vi "Extract Files HTML from SubFolder (Row).vi"(8 "error in (no error)":errorcluster, 10 "SearchFolder":string, 11 "Folder_Mgmt in":refnum<class "Folder_Mgmt.lvclass">) -> (0 "error out":errorcluster, 2 "FolderFiles (Row)":string[](array[string]), 3 "Folder_Mgmt out":refnum<class "Folder_Mgmt.lvclass">)   [LabVIEW 2016, in "Folder_Mgmt.lvclass"]
uses:
  Folder_Mgmt.lvclass
  Folder_Mgmt.lvclass/Folder_Mgmt.ctl
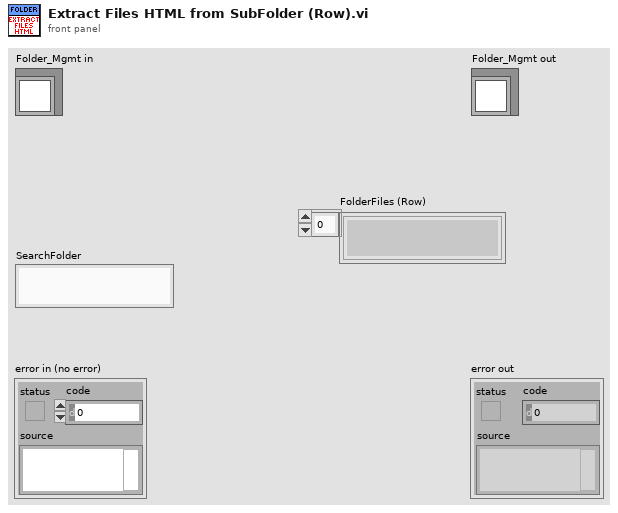
[diagram p1: front panel]
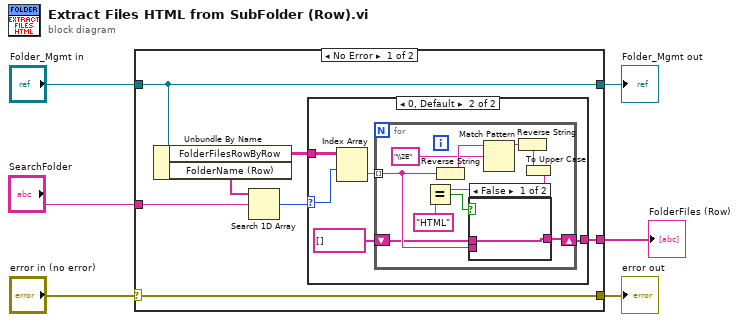
[diagram p0: block diagram]
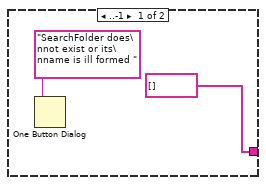
[diagram p2: hidden frame]
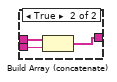
[diagram p3: hidden frame]
diagram:
  n1 = case shown="No Error" "error in (no error)" {
    selector: "error in (no error)" -> [w13 w35]
    tunnel: [w13 w35] -> w5
    tunnel: [w12 w36] -> w3
    tunnel: "Folder_Mgmt in" -> [w12 w36]
    tunnel: [w10 _] -> w2
    tunnel: "SearchFolder" -> [w8 _]
    frame No Error {
      n2 = Unbundle By Name(w12) -> ("FolderFilesRowByRow"=w11:string[][], "FolderName (Row)"=w9:string[])
      n3 = Search 1D Array(1D array=w9, element=w8) -> (index of element=w7:i32)  [unwired: 1 in]
      n4 = case shown="0, Default" w7 {
        selector: w7 -> [_ w19]
        tunnel: w11 -> [_ w20]
        tunnel: [string[] [] ("FolderFilesRowByRow") w16] -> w10
        frame ..-1 {
          n5 = One Button Dialog(message="SearchFolder does\nnot exist or its\nname is ill formed ") -> ()  [unwired: 1 in, 1 out]
        }
        frame 0, Default {
          n6 = Index Array(array=w20, index (row)=w19) -> (element=w18:string[])  [unwired: 1 in]
          n7 = for {
            tunnel: w18 -> [w24] mode=indexing
            shift-right: [w22] -> w16
            shift-left: string[] [] -> [w23]
            n8 = Reverse String(1:w24) -> (0:w30:string)
            n9 = Match Pattern(string=w30, regular expression="\\2E") -> (before substring=w28:string)  [unwired: 1 in, 3 out]
            n10 = Reverse String(1:w28) -> (0:w27:string)
            n11 = To Upper Case(1:w27) -> (0:w21:string)
            n12 = Equal?(x=w21, y="HTML") -> (x = y?=w25:bool)
            n13 = case shown="False" w25 {
              tunnel: w24 -> [_ w34]
              tunnel: w23 -> [w31 w33]
              tunnel: [w31 w32] -> w22
              frame False {
              }
              frame True {
                n14 = Build Array (concatenate)(w33, w34) -> (w32:string[])
              }
            }
          }
        }
      }
    }
    frame Error {
    }
  }
  "error out" <- w5
  "Folder_Mgmt out" <- w3
  "FolderFiles (Row)" <- w2
